vi "LV SCISDK Execute Command.vi"(8 "error in (no error)":errorcluster, 9 "handle":u64, 10 "value":string, 11 "Path":string) -> (0 "error out":errorcluster, 1 "handle out":u64, 3 "function return":i32)   [LabVIEW 2021, in "SciSDK_Labview.lvlib"]
doc: "SCISDKLABVIEW_DLL_API int LV_SCISDK_SetParameterString(char* Path, char* value, void* handle);"
uses:
  SciSDK_Labview.lvlib
  SciSDK_VC++/x64/Debug/SciSDK_Labview.dll
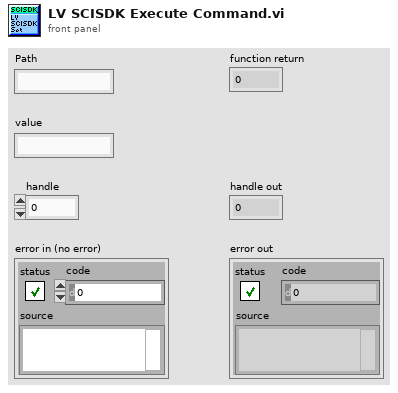
[diagram p1: front panel]
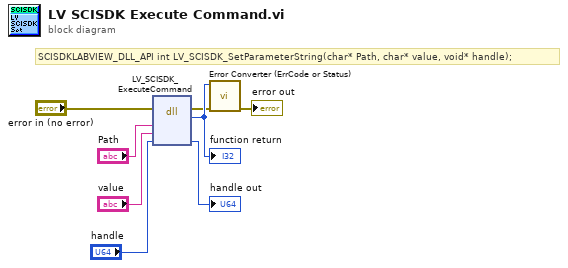
[diagram p0: block diagram]
diagram:
  # "SCISDKLABVIEW_DLL_API int LV_SCISDK_SetParameterString(char* Path, char* value, void* handle);"
  n1 = dll-call lib="C:/git/scisdk/SciSDK_VC++/x64/Debug/SciSDK_Labview.dll" fn="LV_SCISDK_ExecuteCommand"(error in="error in (no error)", "Path"="Path", "value"="value", "handle"="handle") -> (error out=w2:errorcluster, "return type"=w8:i32, "handle"=→"handle out":u64)  [unwired: 4 in, 1 out]
  "function return" <- w8
  n2 = call <userlib>:"Error Converter (ErrCode or Status).vi"("error in (no error)"=w2, "error code"=w8) -> ("error out"=→"error out":errorcluster)  [unwired: 9 in]
